vi "System Time to External Time.vi"(8 "error in (no error)":errorcluster, 9 "ClockID":u8, 10 "System Time":i64, 11 "Clock Convert Map in":T1) -> (0 "error out":errorcluster, 1 "Last Reset Time":i64, 2 "External Time":i64, 3 "Clock Convert Map out":T1)   [LabVIEW 2021, in "Time_CIF_U.lvlib"]
uses:
  Time_CIF_U.lvlib
  Typedef/Clock Conversion Map.ctl
  Typedef/Timestamp Pair.ctl
  Typedef/Errors.ctl
  Errors/Append Error Location.vi
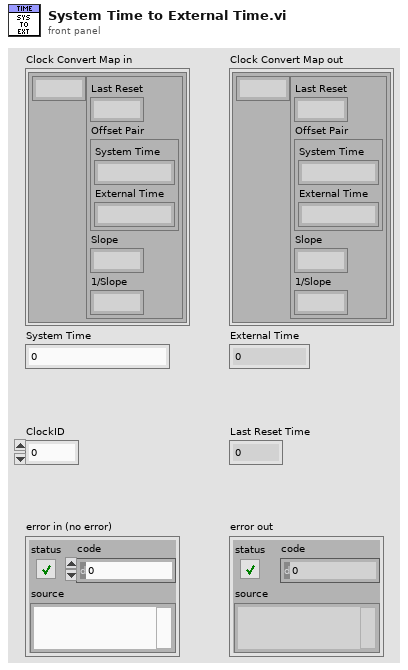
[diagram p1: front panel]
types:
  T1 = typedef "Time_CIF_U.lvlib/Clock Conversion Map.ctl" = map{u8, cluster{"Last Reset":i64, "Offset Pair":T2, "Slope":dbl, "1/Slope":dbl}}
  T2 = typedef "Time_CIF_U.lvlib/Timestamp Pair.ctl" = cluster{"System Time":i64, "External Time":i64}
  T3 = typedef "Time_CIF_U.lvlib/Errors.ctl" = enum16{"Clock ID Match", "Invalid Clock ID", "Long Sleep"}
  T4 = cluster{"Last Reset":i64, "Offset Pair":T2, "Slope":dbl, "1/Slope":dbl}
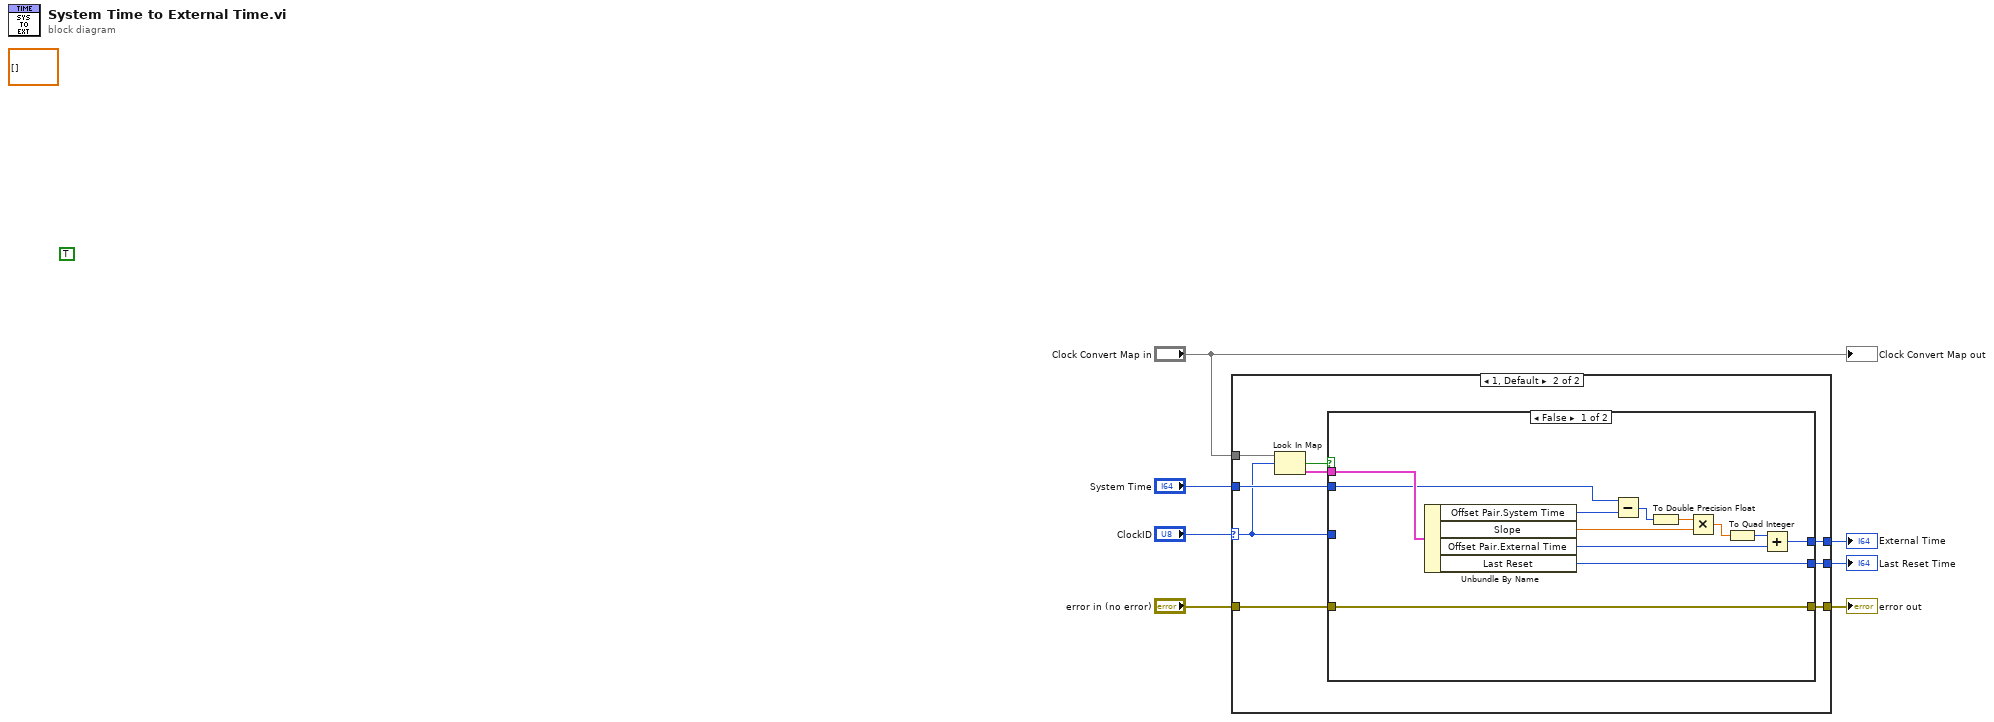
[diagram p0: block diagram]
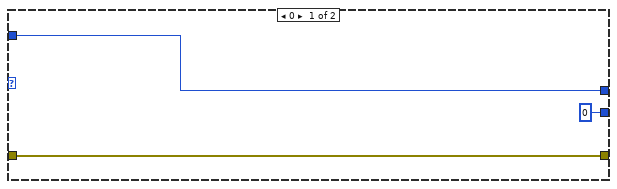
[diagram p2: hidden frame]
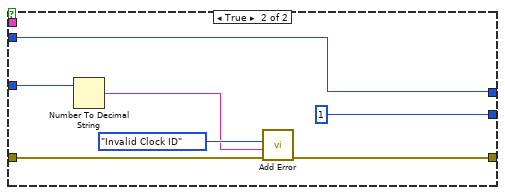
[diagram p3: hidden frame]
diagram:
  (unwired) TRUE
  (unwired) dbl[][] []
  n1 = case shown="1, Default" "ClockID" {
    selector: "ClockID" -> [_ w11]
    tunnel: "System Time" -> [w9 w18]
    tunnel: [w9 w17] -> w6
    tunnel: [i64 0 ("Last Reset") w16] -> w5
    tunnel: "Clock Convert Map in" -> [_ w15]
    tunnel: "error in (no error)" -> [w10 w13]
    tunnel: [w10 w12] -> w2
    frame 0 {
    }
    frame 1, Default {
      n2 = Look In Map(map=w15, key=w11) -> (key not found?=w14:bool, value=w19:T4)  [unwired: 1 in]
      n3 = case shown="False" w14 {
        tunnel: w19 -> [w31 _]
        tunnel: w18 -> [w30 w37]
        tunnel: [w24 w37] -> w17
        tunnel: [w21 i64 1 ("Last Reset")] -> w16
        tunnel: w13 -> [w20 w35]
        tunnel: [w20 w34] -> w12
        tunnel: w11 -> [_ w38]
        frame False {
          n4 = Unbundle By Name(w31) -> ("Offset Pair.System Time"=w23:i64, "Slope"=w29:dbl, "Offset Pair.External Time"=w22:i64, "Last Reset"=w21:i64)
          n5 = Subtract(x=w30, y=w23) -> (x-y=w28:i64)
          n6 = To Double Precision Float(number=w28) -> (double precision float=w27:dbl)
          n7 = Multiply(x=w27, y=w29) -> (x*y=w26:dbl)
          n8 = To Quad Integer(1:w26) -> (0:w25:i64)
          n9 = Add(x=w25, y=w22) -> (x+y=w24:i64)
        }
        frame True {
          n10 = Number To Decimal String(number=w38) -> (decimal integer string=w33:string)  [unwired: 1 in]
          n11 = call "Add Error.vi"("error in (no error)"=w35, "String to Append"=w33, "Error"=Errors."Invalid Clock ID") -> ("error out"=w34:errorcluster)  [unwired: 8 in]
        }
      }
    }
  }
  "External Time" <- w6
  "error out" <- w2
  "Last Reset Time" <- w5
  "Clock Convert Map out" <- "Clock Convert Map in"
